vi "AfterPackageInstallVi.vi"() -> (0 "Error Out":errorcluster)   [LabVIEW 2022 SP3]
doc: "This VI executes immediately after the VI Package is installed. This VI is meant to be selected in the \"Execute the following VI After Package Install\" field of the \"Custom Actions\" page of the VI Package Build Spec (vipb).\n\nThis VI moves the template VIs and CTLs installed by the VI package to a different location.\n\nError handling strategy: Suppress (clear) any/all errors that might occur in this VI."
uses:
  <vilib>/Utility/sysdir.llb/System Directory Type.ctl
panel:
  out "Source Folder Path":path
  out "Destination Folder Path":path
  out "LabVIEW Version Year":string
  # "Development\nControls or indicators that are useful for development or testing, but which are not outputs of the VI."
  # "Input\nInputs to the VI"
  # "Output\nOutputs of the VI"
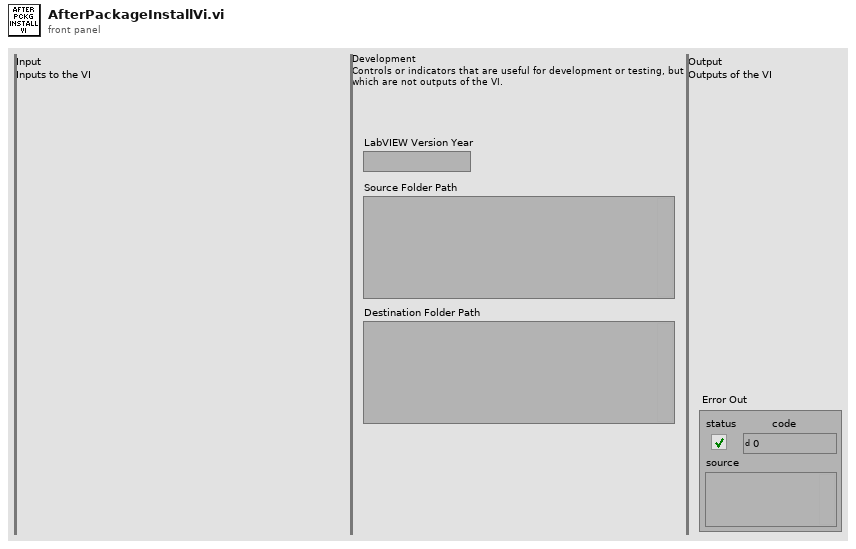
[diagram p1: front panel]
types:
  T1 = typedef "System Directory Type.ctl" = i32
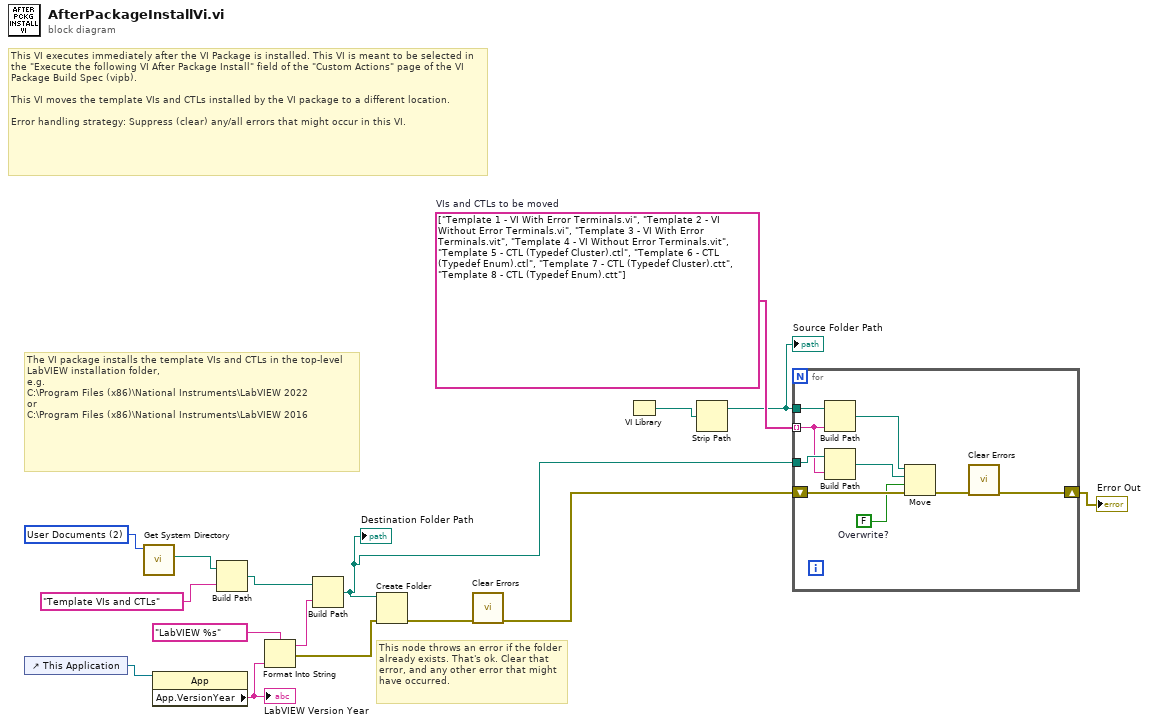
[diagram p0: block diagram]
diagram:
  w15 = T1 2 items=["User Home"=0, "User Desktop"=1, "User Documents"=2, "User Application Data"=3, "User Preferences"=4, "User Temporary"=5, "Public Documents"=6, "Public Application Data"=7, "Public Preferences"=8, "Public Cache"=13, "System Core Libraries"=9, "System Installed Libraries"=10, "Application Files"=11, "Boot Volume Root"=12] ("system directory type")
  w16 = string[] ["Template 1 - VI With Error Terminals.vi", "Template 2 - VI Without Error Terminals.vi", "Template 3 - VI With Error Terminals.vit", "Template 4 - VI Without Error Terminals.vit", "Template 5 - CTL (Typedef Cluster).ctl", "Template 6 - CTL (Typedef Enum).ctl", "Template 7 - CTL (Typedef Cluster).ctt", "Template 8 - CTL (Typedef Enum).ctt"]  # VIs and CTLs to be moved
  # "The VI package installs the template VIs and CTLs in the top-level LabVIEW installation folder,\ne.g. \nC:\\Program Files (x86)\\National Instruments\\LabVIEW 2022\nor\nC:\\Program Files (x86)\\National Instruments\\LabVIEW 2016"
  # "This node throws an error if the folder already exists. That's ok. Clear that error, and any other error that might have occurred."
  # "This VI executes immediately after the VI Package is installed. This VI is meant to be selected in the \"Execute the following VI After Package Install\" field of the \"Custom Actions\" page of the VI Package Build Spec (vipb).\n\nThis VI moves the template VIs and CTLs installed by the VI package to a different location.\n\nError handling strategy: Suppress (clear) any/all errors that might occur in this VI."
  n1 = control-ref of="This Application"() -> (w11:refnum<vi>)
  n2 = call <vilib>:"Get System Directory.vi"("system directory type"=w15) -> ("system directory"=w14:path)  [unwired: 10 in]
  n3 = property class="App"(reference=w11) -> ("App.VersionYear"=w9:string)  [unwired: 1 in, 2 out]
  "LabVIEW Version Year" <- w9
  n4 = Build Path(base path=w14, name or relative path="Template VIs and CTLs") -> (appended path=w13:path)
  n5 = Format Into String(format string="LabVIEW %s", w9) -> (resulting string=w8:string, error out=w7:errorcluster)  [unwired: 2 in]
  n6 = Build Path(base path=w13, name or relative path=w8) -> (appended path=w3:path)
  "Destination Folder Path" <- w3
  n7 = Create Folder(path (use dialog)=w3, error in=w7) -> (error out=w6:errorcluster)  [unwired: 1 in, 2 out]
  n8 = call <vilib>:"Clear Errors.vi"("error in (no error)"=w6) -> ("error out"=w4:errorcluster)  [unwired: 5 in, 1 out]
  n9 = VI Library() -> (path=w5:path)
  n10 = Strip Path(path=w5) -> (stripped path=w1:path)  [unwired: 1 out]
  "Source Folder Path" <- w1
  n11 = for {
    tunnel: w16 -> [w21] mode=indexing
    tunnel: w1 -> [w25]
    tunnel: w3 -> [w22]
    shift-right: [w17] -> w2
    shift-left: w4 -> [w23]
    w19 = FALSE  # Overwrite?
    n12 = Build Path(base path=w25, name or relative path=w21) -> (appended path=w24:path)
    n13 = Build Path(base path=w22, name or relative path=w21) -> (appended path=w20:path)
    n14 = Move(source path=w24, error in=w23, 9:w19, 10:w20) -> (error out=w18:errorcluster)  [unwired: 1 in, 2 out]
    n15 = call <vilib>:"Clear Errors.vi"("error in (no error)"=w18) -> ("error out"=w17:errorcluster)  [unwired: 5 in, 1 out]
  }
  "Error Out" <- w2
